vi "Table Cell.vi"(4 "Colspan (0)":i32, 5 "Rowspan (0)":i32, 6 "Class (\"\")":string, 8 "Cell String (\"\")":string, 9 "Previous HTML in":string) -> (3 "HTML out":string)   [LabVIEW 2011]
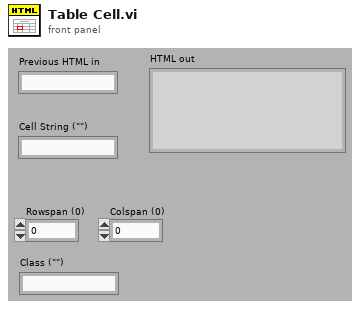
[diagram p1: front panel]
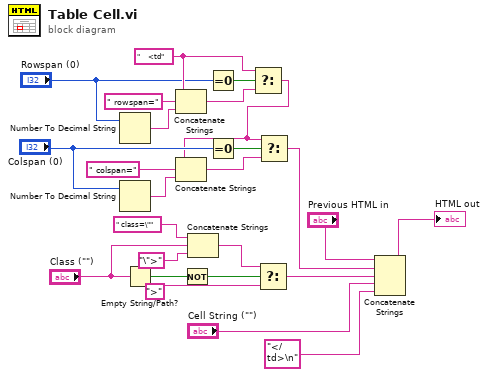
[diagram p0: block diagram]
diagram:
  w11 = "    <td"
  n1 = Number To Decimal String(number="Rowspan (0)") -> (decimal integer string=w8:string)  [unwired: 1 out]
  n2 = Number To Decimal String(number="Colspan (0)") -> (decimal integer string=w4:string)  [unwired: 1 out]
  n3 = Empty String/Path?(string/path="Class (\"\")") -> (empty?=w21:bool)
  n4 = Concatenate Strings(w11, " rowspan=", w8) -> (w12:string)
  n5 = Not(x=w21) -> (.not. x?=w17:bool)
  n6 = Concatenate Strings(" class=\"", "Class (\"\")", "\">") -> (w19:string)
  n7 = Equal To 0?(x="Rowspan (0)") -> (x = 0?=w13:bool)
  n8 = Equal To 0?(x="Colspan (0)") -> (x = 0?=w5:bool)
  n9 = Select(t=w11, s=w13, f=w12) -> (s? t:f=w1:string)
  n10 = Concatenate Strings(w1, " colspan=", w4) -> (w6:string)
  n11 = Select(t=w19, s=w17, f=">") -> (s? t:f=w14:string)
  n12 = Select(t=w1, s=w5, f=w6) -> (s? t:f=w2:string)
  n13 = Concatenate Strings("Previous HTML in", w2, w14, "Cell String (\"\")", "</td>\n") -> (→"HTML out":string)
